vi "Read File.vi"(8 "error in":errorcluster, 11 "Data Cluster In":T1={"UI Reference"={"All Ctrl's Label's"=[], "ChannelListTree"=refnum, "All Object Ref"=[]}, "Tree Selection"={"Selected Channel"="", "Selected Interface"="", "Selected HW"="", "Tree Root Name"="", "Selected Module"=""}, "Selected File Path"=path "", "Selected HW"={"Slctd Hw Name"=[], "Slctd HW IP"=[]}, "Channel Config Path"=path "", "Interface Data"={"DO Channel's"=[]}, "General Info's"={"Idnentification name"=""}, "Status"="", "Channel Type's"={"Channel Type"=enum."Voltage", "Sub-Type"=enum."Pressure"}, "This VI"=refnum, "Hardware Information "=variant(variant[] [])}) -> (0 "error out":errorcluster, 3 "Data Cluster Out":T1={"UI Reference"={"All Ctrl's Label's"=[], "ChannelListTree"=refnum, "All Object Ref"=[]}, "Tree Selection"={"Selected Channel"="", "Selected Interface"="", "Selected HW"="", "Tree Root Name"="", "Selected Module"=""}, "Selected File Path"=path "", "Selected HW"={"Slctd Hw Name"=[], "Slctd HW IP"=[]}, "Channel Config Path"=path "", "Interface Data"={"DO Channel's"=[]}, "General Info's"={"Idnentification name"=""}, "Status"="", "Channel Type's"={"Channel Type"=enum."Voltage", "Sub-Type"=enum."Pressure"}, "This VI"=refnum, "Hardware Information "=variant(variant[] [])})   [LabVIEW 2021, in "Configuration.lvlib"]
doc: "<b>Note:</b> This VI was modified by the <b>Validate DQMH Module</b> tool to turn off automatic error handling."
uses:
  Configuration.lvlib
  Module Data--cluster.ctl
  Host-Control's/Configuration UI Reference.ctl
  DO Channel's.ctl
  Config-Channel Type.ctl
  Channel Sub-Type.ctl
  All Interface Data.ctl
  Analog Input Single Channel Data--Cluster.ctl
  Analog Output/Controls/AO Timing Cluster.ctl
  <vilib>/Utility/xml.llb/Read From XML File.vi
  <vilib>/Utility/xml.llb/Read From XML File(string).vi
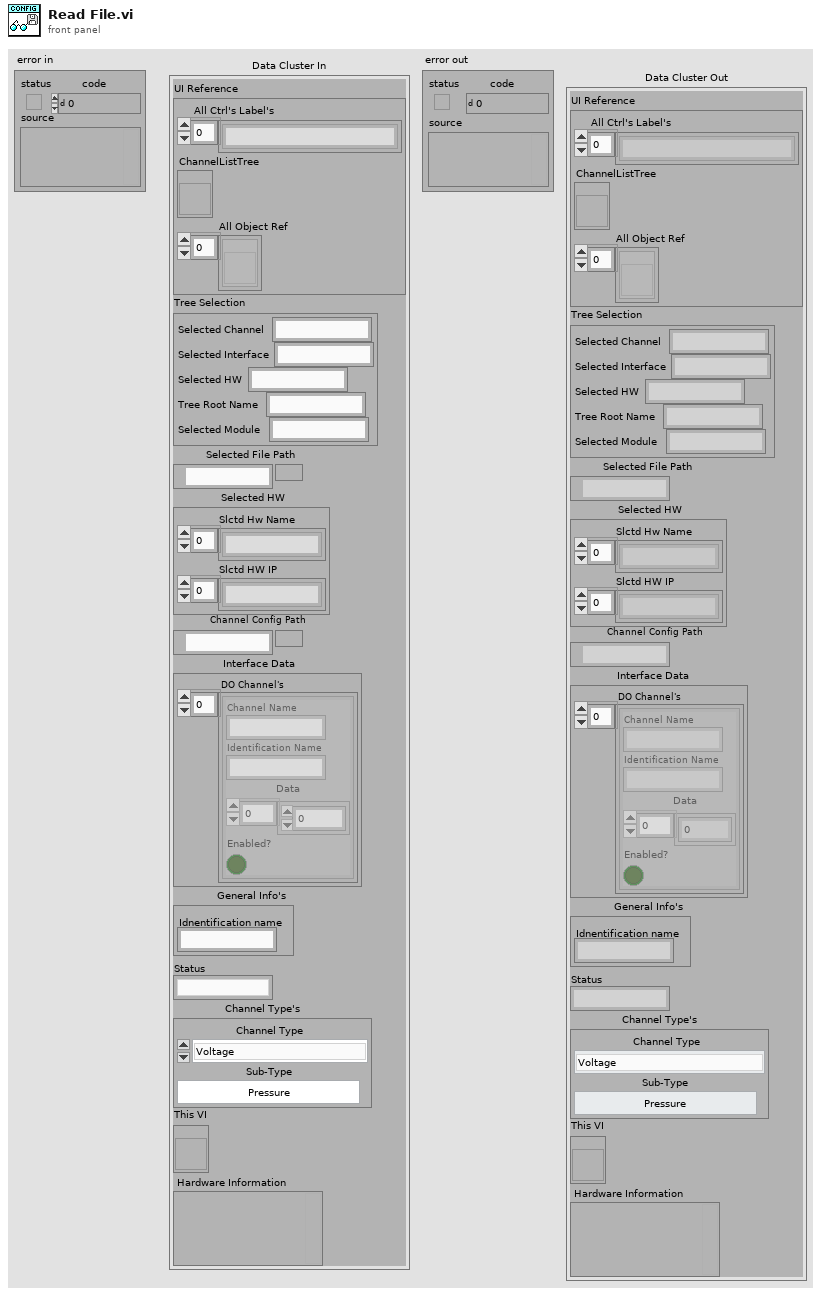
[diagram p1: front panel]
types:
  T1 = typedef "Configuration.lvlib/Module Data--cluster.ctl" = cluster{"UI Reference":T2, "Tree Selection":cluster{"Selected Channel":string, "Selected Interface":string, "Selected HW":string, "Tree Root Name":string, "Selected Module":string}, "Selected File Path":path, "Selected HW":cluster{"Slctd Hw Name":string[], "Slctd HW IP":string[]}, "Channel Config Path":path, "Interface Data":cluster{"DO Channel's":T3}, "General Info's":cluster{"Idnentification name":string}, "Status":string, "Channel Type's":cluster{"Channel Type":T4, "Sub-Type":T5}, "This VI":refnum<vi>, "Hardware Information ":variant}
  T2 = typedef "Configuration UI Reference.ctl" = cluster{"All Ctrl's Label's":string[], "ChannelListTree":refnum<vi>, "All Object Ref":refnum<vi>[]}
  T3 = typedef "Configuration.lvlib/DO Channel's.ctl" = cluster{"Channel Name":string, "Identification Name":string, "Data":u8[], "Enabled?":bool}[]
  T4 = typedef "Configuration.lvlib/Config-Channel Type.ctl" = enum16{"Voltage", "Current", "Thermocouple", "Acclerometer"}
  T5 = typedef "Configuration.lvlib/Channel Sub-Type.ctl" = enum16{"None", "Pressure", "Force"}
  T6 = typedef "Configuration.lvlib/All Interface Data.ctl" = cluster{"DI Config Data":T3, "DO Config Data":T3, "AI Config Data's":cluster{"Module Name":string, "AI Channel's Data":T7[], "Analog Input Timing":T8}[]}
  T7 = typedef "Configuration.lvlib/Analog Input Single Channel Data--Cluster.ctl" = cluster{"Channel Name":string, "Identification Name":string, "Channel Type":T4, "Sub-Type":T5, "Data":string, "Enabled?":bool}
  T8 = typedef "AO Timing Cluster.ctl" = cluster{"samples per channel":i32, "sample mode":i32, "Sampling Rate":dbl}
  T9 = cluster{"Channel Name":string, "Identification Name":string, "Data":u8[], "Enabled?":bool}
  T10 = cluster{"Module Name":string, "AI Channel's Data":T7[], "Analog Input Timing":T8}[]
  T11 = cluster{"Module Name":string, "AI Channel's Data":T7[], "Analog Input Timing":T8}
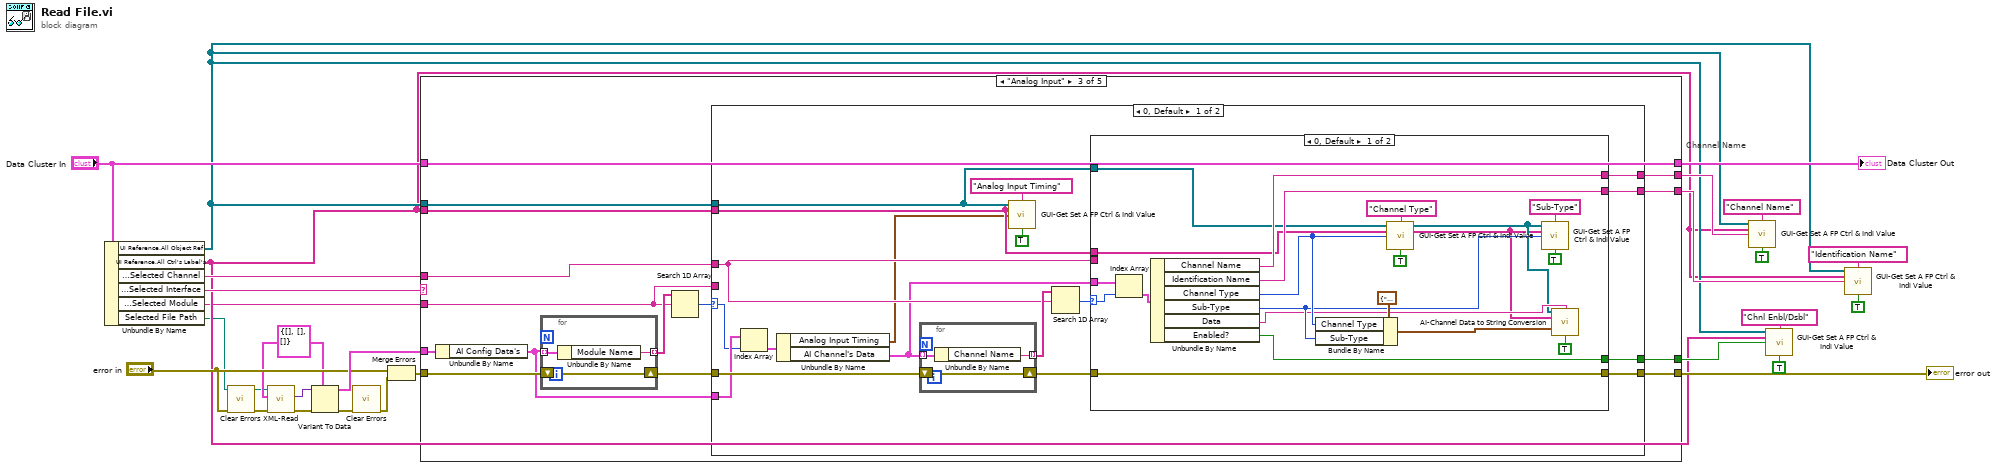
[diagram p0: block diagram]
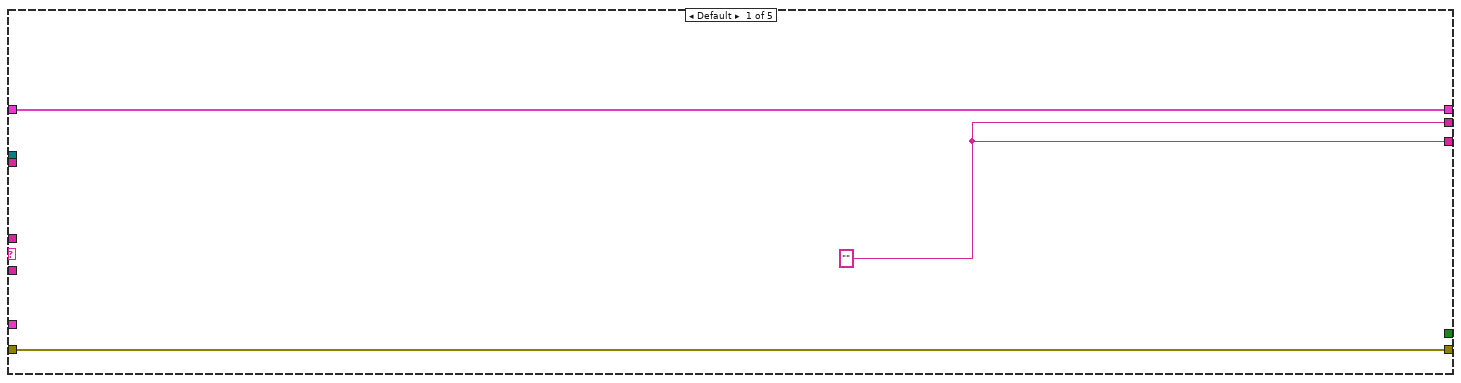
[diagram p2: hidden frame]
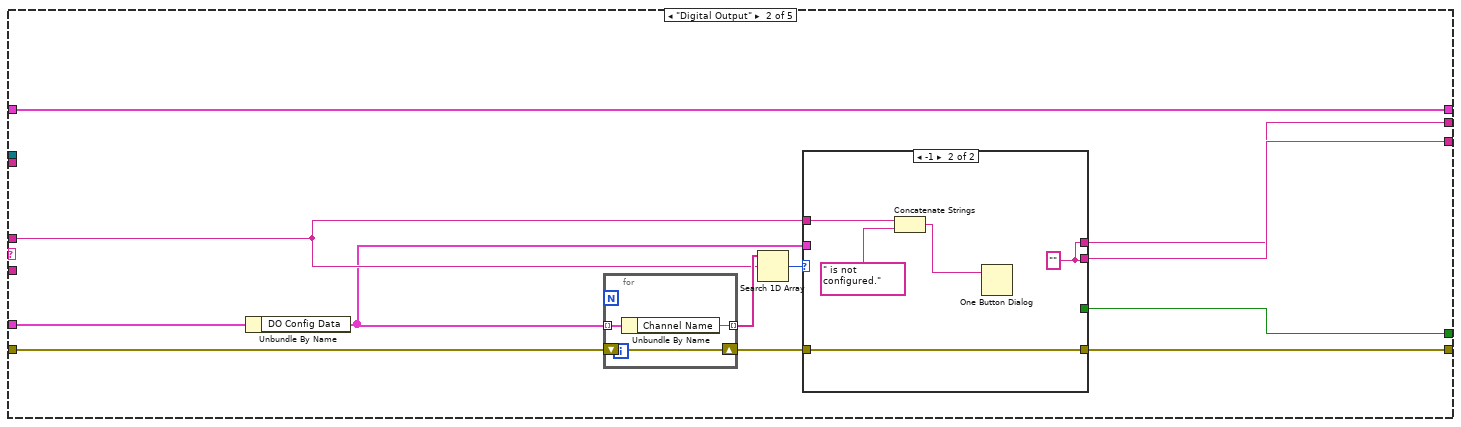
[diagram p3: hidden frame]
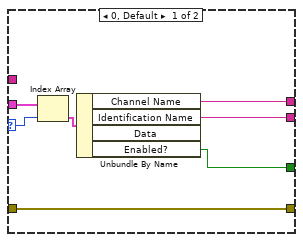
[diagram p4: hidden frame]
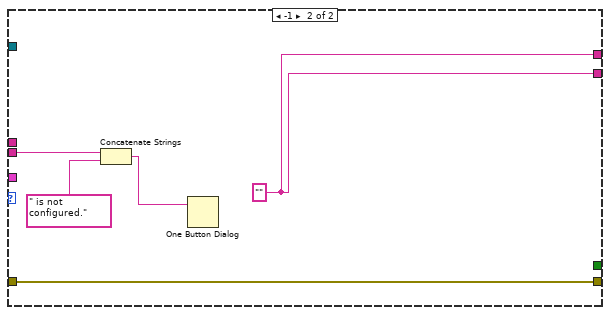
[diagram p5: hidden frame]
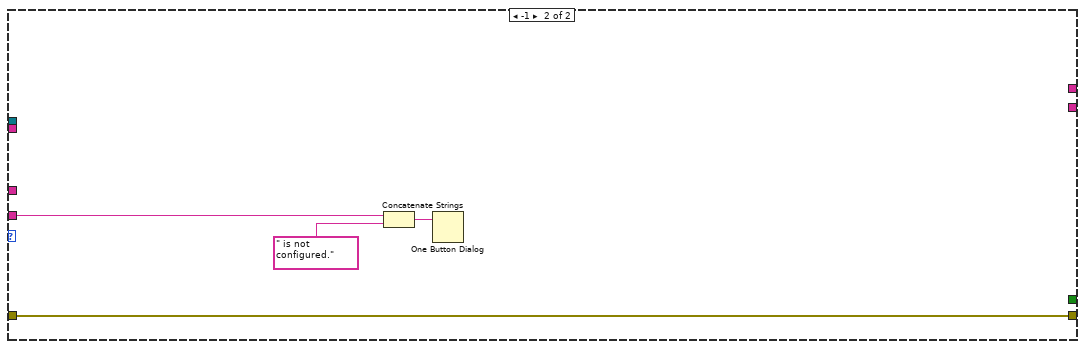
[diagram p6: hidden frame]
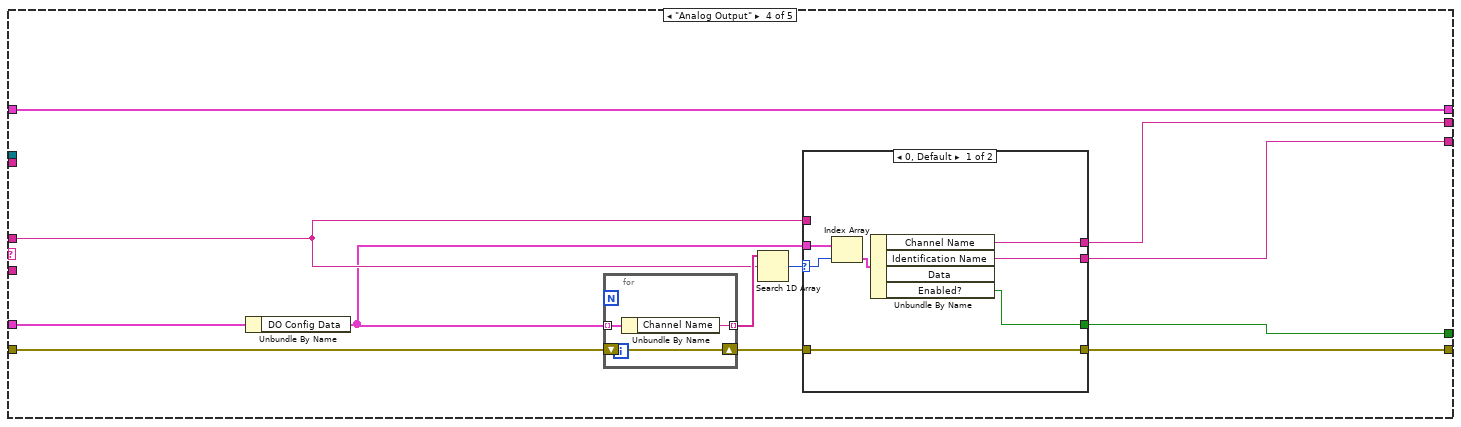
[diagram p7: hidden frame]
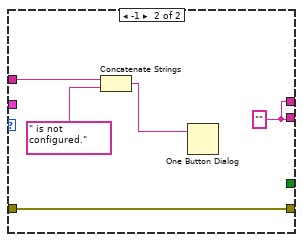
[diagram p8: hidden frame]
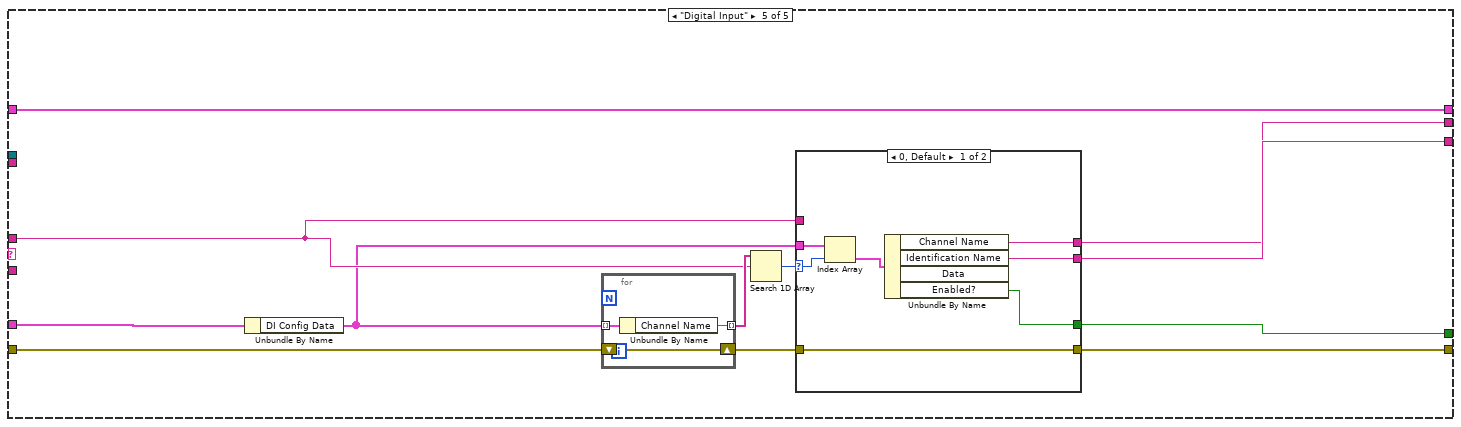
[diagram p9: hidden frame]
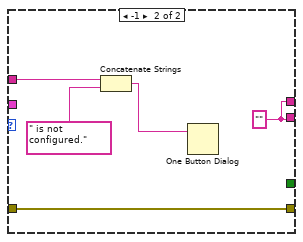
[diagram p10: hidden frame]
diagram:
  w6 = T6 {"DI Config Data"=[], "DO Config Data"=[], "AI Config Data's"=[]} ("Interface Data")
  # "Channel Name"
  n1 = Unbundle By Name("Data Cluster In") -> ("UI Reference.All Object Ref"=w8:refnum<vi>[], "UI Reference.All Ctrl's Label's"=w7:string[], "Tree Selection.Selected Channel"=w23:string, "Tree Selection.Selected Interface"=w27:string, "Tree Selection.Selected Module"=w1:string, "Selected File Path"=w2:path)
  n2 = call <vilib>:"Clear Errors.vi"("error in (no error)"="error in") -> ("error out"=w5:errorcluster)  [unwired: 5 in, 1 out]
  n3 = call "XML-Read.vi"("error in (no error)"=w5, "Data"=w6, "XML File Path"=w2) -> ("error out"=w4:errorcluster, "Data Out"=w3:variant)  [unwired: 6 in, 1 out]
  n4 = Variant To Data(error in=w4, type=w6, Variant=w3) -> (data=w19:T6, error out=w21:errorcluster)
  n5 = call <vilib>:"Clear Errors.vi"("error in (no error)"=w21) -> ("error out"=w22:errorcluster)  [unwired: 5 in, 1 out]
  n6 = Merge Errors("error in", w22) -> (w20:errorcluster)
  n7 = case shown="\"Analog Input\"" w27 {
    tunnel: w20 -> [w30 w33 w63 w127 w154]
    tunnel: [w30 w37 w69 w131 w159] -> w26
    tunnel: [w29 w42 w72 w136 w163] -> w25
    tunnel: "Data Cluster In" -> [w29 w42 w72 w136 w163]
    tunnel: w23 -> [_ w38 w70 w132 w155]
    tunnel: [w28 w40 w71 w134 w161] -> w14
    tunnel: [w28 w35 w68 w129 w157] -> w15
    tunnel: w19 -> [_ w34 w64 w128 w156]
    tunnel: [_ w31 w67 w125 w152] -> w13
    tunnel: w8 -> [_ _ w66 _ _]
    tunnel: w7 -> [_ _ w65 _ _]
    tunnel: w1 -> [_ _ w59 _ _]
    frame Default {
      w28 = "" ("Identification Name")
    }
    frame "Digital Output" {
      n8 = Unbundle By Name(w34) -> ("DO Config Data"=w32:T3)
      n9 = for {
        tunnel: w32 -> [w56] mode=indexing
        shift-right: [w57] -> w36
        shift-left: w33 -> [w57]
        tunnel: [w55] -> w41 mode=indexing
        n10 = Unbundle By Name(w56) -> ("Channel Name"=w55:string)
      }
      n11 = Search 1D Array(1D array=w41, element=w38) -> (index of element=w39:i32)  [unwired: 1 in]
      n12 = case shown="-1" w39 {
        selector: w39 -> [w46 _]
        tunnel: w32 -> [w49 _]
        tunnel: [w47 w50] -> w40
        tunnel: w38 -> [_ w53]
        tunnel: [w45 w54] -> w37
        tunnel: w36 -> [w45 w54]
        tunnel: [w44 w50] -> w35
        tunnel: [w43 _] -> w31
        frame 0, Default {
          n13 = Index Array(array=w49, index=w46) -> (element=w48:T9)
          n14 = Unbundle By Name(w48) -> ("Channel Name"=w44:string, "Identification Name"=w47:string, "Enabled?"=w43:bool)  [unwired: 1 out]
        }
        frame -1 {
          w50 = "" ("Identification Name")
          n15 = Concatenate Strings(w53, " is not configured." ("Identification Name")) -> (w51:string)
          n16 = One Button Dialog(message=w51) -> ()  [unwired: 1 in, 1 out]
        }
      }
    }
    frame "Analog Input" {
      n17 = Unbundle By Name(w64) -> ("AI Config Data's"=w58:T10)
      n18 = for {
        tunnel: w58 -> [w123] mode=indexing
        shift-right: [w124] -> w62
        shift-left: w63 -> [w124]
        tunnel: [w122] -> w61 mode=indexing
        n19 = Unbundle By Name(w123) -> ("Module Name"=w122:string)
      }
      n20 = Search 1D Array(1D array=w61, element=w59) -> (index of element=w60:i32)  [unwired: 1 in]
      n21 = case shown="0, Default" w60 {
        selector: w60 -> [w76 _]
        tunnel: [w89 _] -> w71
        tunnel: w70 -> [w87 _]
        tunnel: [w86 w118] -> w69
        tunnel: [w84 _] -> w68
        tunnel: [w83 _] -> w67
        tunnel: w66 -> [w80 _]
        tunnel: w65 -> [w79 _]
        tunnel: w62 -> [w78 w118]
        tunnel: w59 -> [_ w119]
        tunnel: w58 -> [w77 _]
        frame 0, Default {
          n22 = Index Array(array=w77, index=w76) -> (element=w75:T11)
          n23 = Unbundle By Name(w75) -> ("Analog Input Timing"=w74:T8, "AI Channel's Data"=w73:T7[])
          n24 = for {
            shift-right: [w93] -> w85
            shift-left: w78 -> [w93]
            tunnel: [w92] -> w90 mode=indexing
            tunnel: w73 -> [w91] mode=indexing
            n25 = Unbundle By Name(w91) -> ("Channel Name"=w92:string)
          }
          n26 = call "GUI-Get Set A FP Ctrl & Indi Value.vi"("All Object Ref"=w80, "Label"="Analog Input Timing" ("Label In"), "All Object Label"=w79, "Ctrl Value In"=w74, "Set(F)"=TRUE) -> ()  [unwired: 7 in, 4 out]
          n27 = Search 1D Array(1D array=w90, element=w87) -> (index of element=w88:i32)  [unwired: 1 in]
          n28 = case shown="0, Default" w88 {
            selector: w88 -> [w109 _]
            tunnel: w73 -> [w112 _]
            tunnel: [w110 w113] -> w89
            tunnel: w87 -> [_ w116]
            tunnel: [w108 w117] -> w86
            tunnel: w85 -> [w108 w117]
            tunnel: [w107 w113] -> w84
            tunnel: [w106 _] -> w83
            tunnel: w80 -> [w95 _]
            tunnel: w79 -> [w94 _]
            frame 0, Default {
              n29 = Index Array(array=w112, index=w109) -> (element=w111:T7)
              n30 = Unbundle By Name(w111) -> ("Channel Name"=w107:string, "Identification Name"=w110:string, "Channel Type"=w100:T4, "Sub-Type"=w99:T5, "Data"=w96:string, "Enabled?"=w106:bool)
              n31 = Bundle By Name(cluster=cluster{"Channel Type":T4, "Sub-Type":T5} {"Channel Type"=enum."Voltage", "Sub-Type"=enum."None"} ("Channel Types'"), "Channel Type"=w100, "Sub-Type"=w99) -> (w98:cluster{"Channel Type":T4, "Sub-Type":T5})
              n32 = call "GUI-Get Set A FP Ctrl & Indi Value.vi"("All Object Ref"=w95, "Label"="Channel Type" ("Label In"), "All Object Label"=w94, "Ctrl Value In"=w100, "Set(F)"=TRUE) -> ()  [unwired: 7 in, 4 out]
              n33 = call "GUI-Get Set A FP Ctrl & Indi Value.vi"("All Object Ref"=w95, "Label"="Sub-Type" ("Label In"), "All Object Label"=w94, "Ctrl Value In"=w99, "Set(F)"=TRUE) -> ()  [unwired: 7 in, 4 out]
              n34 = call "AI-Channel Data to String Conversion.vi"("All Object Ref"=w95, "XML String In"=w96, "All Object Label"=w94, "Channel Types'"=w98, "Write to Ctrl (F)"=TRUE) -> ()  [unwired: 10 in, 1 out]
            }
            frame -1 {
              w113 = "" ("Identification Name")
              n35 = Concatenate Strings(w116, " is not configured." ("Identification Name")) -> (w114:string)
              n36 = One Button Dialog(message=w114) -> ()  [unwired: 1 in, 1 out]
            }
          }
        }
        frame -1 {
          n37 = Concatenate Strings(w119, " is not configured." ("Identification Name")) -> (w120:string)
          n38 = One Button Dialog(message=w120) -> ()  [unwired: 1 in, 1 out]
        }
      }
    }
    frame "Analog Output" {
      n39 = Unbundle By Name(w128) -> ("DO Config Data"=w126:T3)
      n40 = for {
        tunnel: w126 -> [w150] mode=indexing
        shift-right: [w151] -> w130
        shift-left: w127 -> [w151]
        tunnel: [w149] -> w135 mode=indexing
        n41 = Unbundle By Name(w150) -> ("Channel Name"=w149:string)
      }
      n42 = Search 1D Array(1D array=w135, element=w132) -> (index of element=w133:i32)  [unwired: 1 in]
      n43 = case shown="0, Default" w133 {
        selector: w133 -> [w140 _]
        tunnel: w126 -> [w143 _]
        tunnel: [w141 w144] -> w134
        tunnel: w132 -> [_ w147]
        tunnel: [w139 w148] -> w131
        tunnel: w130 -> [w139 w148]
        tunnel: [w138 w144] -> w129
        tunnel: [w137 _] -> w125
        frame 0, Default {
          n44 = Index Array(array=w143, index=w140) -> (element=w142:T9)
          n45 = Unbundle By Name(w142) -> ("Channel Name"=w138:string, "Identification Name"=w141:string, "Enabled?"=w137:bool)  [unwired: 1 out]
        }
        frame -1 {
          w144 = "" ("Identification Name")
          n46 = Concatenate Strings(w147, " is not configured." ("Identification Name")) -> (w145:string)
          n47 = One Button Dialog(message=w145) -> ()  [unwired: 1 in, 1 out]
        }
      }
    }
    frame "Digital Input" {
      n48 = Unbundle By Name(w156) -> ("DI Config Data"=w153:T3)
      n49 = for {
        tunnel: w153 -> [w176] mode=indexing
        shift-right: [w178] -> w158
        shift-left: w154 -> [w178]
        tunnel: [w177] -> w162 mode=indexing
        n50 = Unbundle By Name(w176) -> ("Channel Name"=w177:string)
      }
      n51 = Search 1D Array(1D array=w162, element=w155) -> (index of element=w160:i32)  [unwired: 1 in]
      n52 = case shown="0, Default" w160 {
        selector: w160 -> [w170 _]
        tunnel: w153 -> [w168 _]
        tunnel: [w165 w171] -> w161
        tunnel: w155 -> [_ w174]
        tunnel: [w169 w175] -> w159
        tunnel: w158 -> [w169 w175]
        tunnel: [w166 w171] -> w157
        tunnel: [w164 _] -> w152
        frame 0, Default {
          n53 = Index Array(array=w168, index=w170) -> (element=w167:T9)
          n54 = Unbundle By Name(w167) -> ("Channel Name"=w166:string, "Identification Name"=w165:string, "Enabled?"=w164:bool)  [unwired: 1 out]
        }
        frame -1 {
          w171 = "" ("Identification Name")
          n55 = Concatenate Strings(w174, " is not configured." ("Identification Name")) -> (w172:string)
          n56 = One Button Dialog(message=w172) -> ()  [unwired: 1 in, 1 out]
        }
      }
    }
  }
  "error out" <- w26
  "Data Cluster Out" <- w25
  n57 = call "GUI-Get Set A FP Ctrl & Indi Value.vi"("All Object Ref"=w8, "Label"="Channel Name" ("Label In"), "All Object Label"=w7, "Ctrl Value In"=w15, "Set(F)"=TRUE) -> ()  [unwired: 7 in, 4 out]
  n58 = call "GUI-Get Set A FP Ctrl & Indi Value.vi"("All Object Ref"=w8, "Label"="Chnl Enbl/Dsbl" ("Label In"), "All Object Label"=w7, "Ctrl Value In"=w13, "Set(F)"=TRUE) -> ()  [unwired: 7 in, 4 out]
  n59 = call "GUI-Get Set A FP Ctrl & Indi Value.vi"("All Object Ref"=w8, "Label"="Identification Name" ("Label In"), "All Object Label"=w7, "Ctrl Value In"=w14, "Set(F)"=TRUE) -> ()  [unwired: 7 in, 4 out]
